vi "Untitled 2.vi"() -> ()   [LabVIEW 2015]
panel:
  out "Numeric":i32
  in  "stop":bool
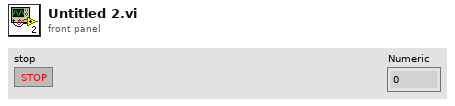
[diagram p1: front panel]
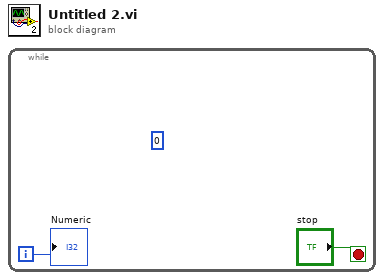
[diagram p0: block diagram]
diagram:
  n1 = while {
    i -> [w1]
    stop <- "stop" stop-if-true
    (unwired) 0
    "Numeric" <- w1
  }
